vi "Read Times Repeat.vi"(8 "error in (no error)":errorcluster, 11 "RepeatingDirector in":refnum<class "RepeatingDirector.lvclass">) -> (0 "error out":errorcluster, 2 "Times Repeat":u32=1 min=1 step=1, 3 "RepeatingDirector out":refnum<class "RepeatingDirector.lvclass">)   [LabVIEW 2023, in "HAF.lvlib" / "RepeatingDirector.lvclass"]
doc: "Returns the number of times the Commands should be repeated."
uses:
  RepeatingDirector.lvclass
  RepeatingDirector.lvclass/RepeatingDirector.ctl
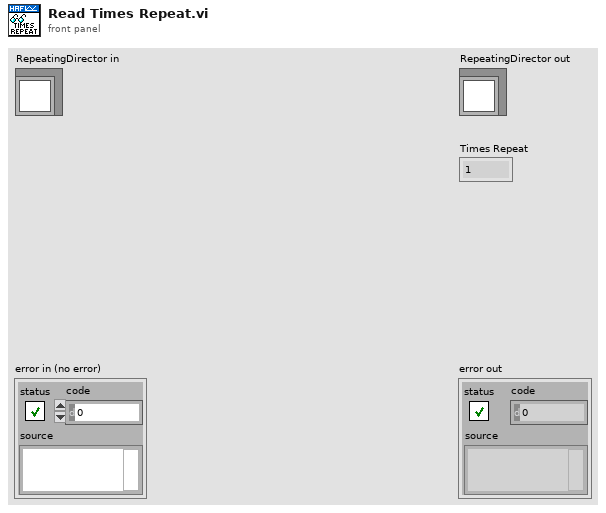
[diagram p1: front panel]
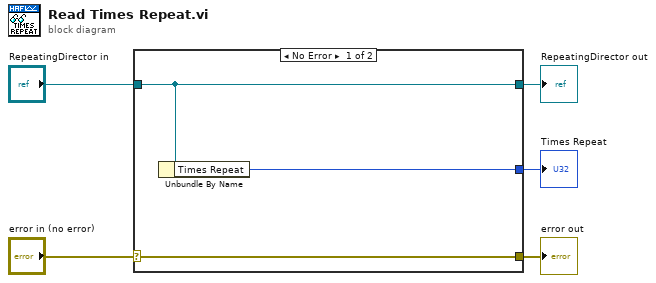
[diagram p0: block diagram]
diagram:
  n1 = case shown="No Error" "error in (no error)" {
    selector: "error in (no error)" -> [w8 w9]
    tunnel: [w8 w9] -> w4
    tunnel: [w7 w10] -> w2
    tunnel: "RepeatingDirector in" -> [w7 w10]
    tunnel: [w6 _] -> w1
    frame No Error {
      n2 = Unbundle By Name(w7) -> ("Times Repeat"=w6:u32)
    }
    frame Error {
    }
  }
  "error out" <- w4
  "RepeatingDirector out" <- w2
  "Times Repeat" <- w1
